vi "send delta to waveform.vi"(8 "error in (no error)":errorcluster, 11 "LineCCD in":refnum<class "LineCCD.lvclass">) -> (0 "error out":errorcluster, 3 "LineCCD out":refnum<class "LineCCD.lvclass">)   [LabVIEW 2012, in "LineCCD.lvclass"]
uses:
  LineCCD.lvclass
  <vilib>/Distrio/Murmex/GenericMessage/GenericMessage.lvclass
  LineCCD.lvclass/LineCCD.ctl
  <vilib>/Distrio/Murmex/Message/Message.lvclass
  <vilib>/Distrio/Murmex/Murmex/Murmex.lvclass
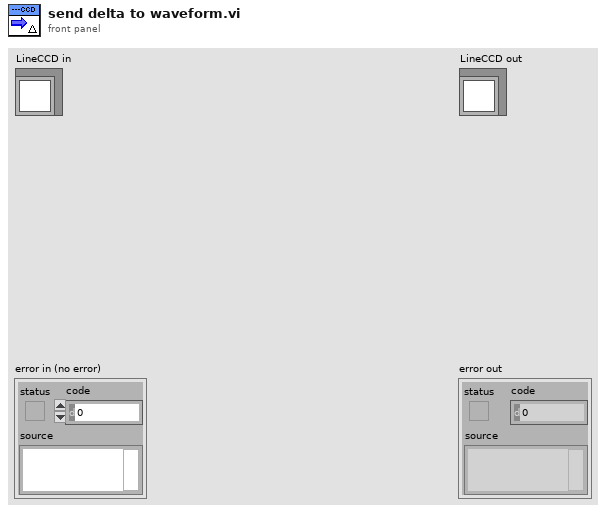
[diagram p1: front panel]
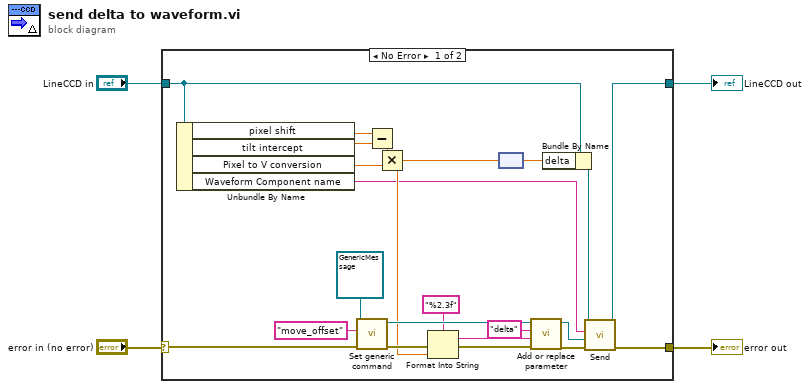
[diagram p0: block diagram]
diagram:
  n1 = case shown="No Error" "error in (no error)" {
    selector: "error in (no error)" -> [w6 w28]
    tunnel: [w5 w28] -> w3
    tunnel: [w10 w27] -> w1
    tunnel: "LineCCD in" -> [w22 w27]
    frame No Error {
      n2 = Unbundle By Name(w22) -> ("pixel shift"=w26:dbl, "tilt intercept"=w25:dbl, "Pixel to V conversion"=w24:dbl, "Waveform Component name"=w9:string)
      n3 = call <vilib>:"Set generic command.vi"("error in (no error)"=w6, "generic command"="move_offset", "GenericMessage in"=refnum<class "GenericMessage.lvclass"> refnum ("Message in")) -> ("error out"=w16:errorcluster, "GenericMessage out"=w18:refnum<class "GenericMessage.lvclass">)  [unwired: 7 in]
      n4 = Subtract(x=w26, y=w25) -> (x-y=w23:dbl)
      n5 = Multiply(x=w23, y=w24) -> (x*y=w13:dbl)
      n6 = Format Into String(format string="%2.3f", error in=w16, w13) -> (resulting string=w8:string, error out=w15:errorcluster)  [unwired: 1 in]
      n7 = node(w13) -> (w21:dbl[unit])
      n8 = call <vilib>:"Add or replace parameter.vi"("error in (no error)"=w15, "value"=w8, "name"="delta", "Message in"=w18) -> ("error out"=w12:errorcluster, "Message out"=w7:refnum<class "GenericMessage.lvclass">)  [unwired: 6 in]
      n9 = Bundle By Name(cluster=w22, "delta"=w21) -> (w11:refnum<class "LineCCD.lvclass">)
      n10 = call <vilib>:"Send.vi"("error in (no error)"=w12, "Message"=w7, "recipient"=w9, "Murmex in"=w11) -> ("error out"=w5:errorcluster, "Murmex out"=w10:refnum<class "LineCCD.lvclass">)  [unwired: 6 in]
    }
    frame Error {
    }
  }
  "error out" <- w3
  "LineCCD out" <- w1
